vi "comunicación_arduino.vi"() -> ()   [LabVIEW 2026]
uses:
  <vilib>/Instr/_visa.llb/VISA Configure Serial Port (Instr).vi
  <vilib>/Utility/file.llb/Write Delimited Spreadsheet (string).vi
panel:
  out "LED de Histéresis":bool
  in  "Histeresis":dbl
  out "Rango de umbral":bool
  in  "Umbral minimo":dbl
  in  "Umbral maximo":dbl
  in  "Guardar datos":bool
  out "Temperatura minima":dbl
  out "Temperatura maxima":dbl
  out "Waveform Chart":cluster{dbl, dbl, dbl}(graph)
  out "Valor sin filtrar":dbl
  in  "Valor filtrado":bool
  out "Valor filtrado":dbl
  in  "data bits (8)":u16=8 min=5 max=8 step=1
  in  "baud rate (9600)":u32=9600
  out "Dato resivido":string
  in  "Dato a enviar":string
  in  "stop":bool
  in  "Escritura":bool
  in  "Lectura":bool
  in  "VISA resource name":refnum<visa-resource-name>
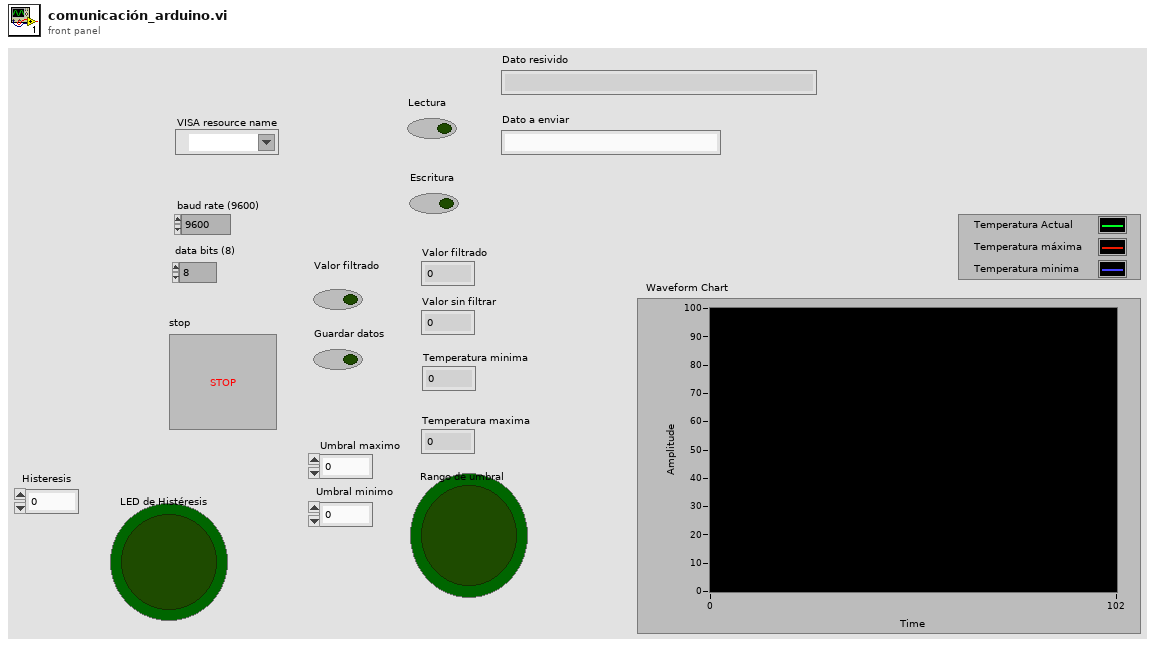
[diagram p1: front panel]
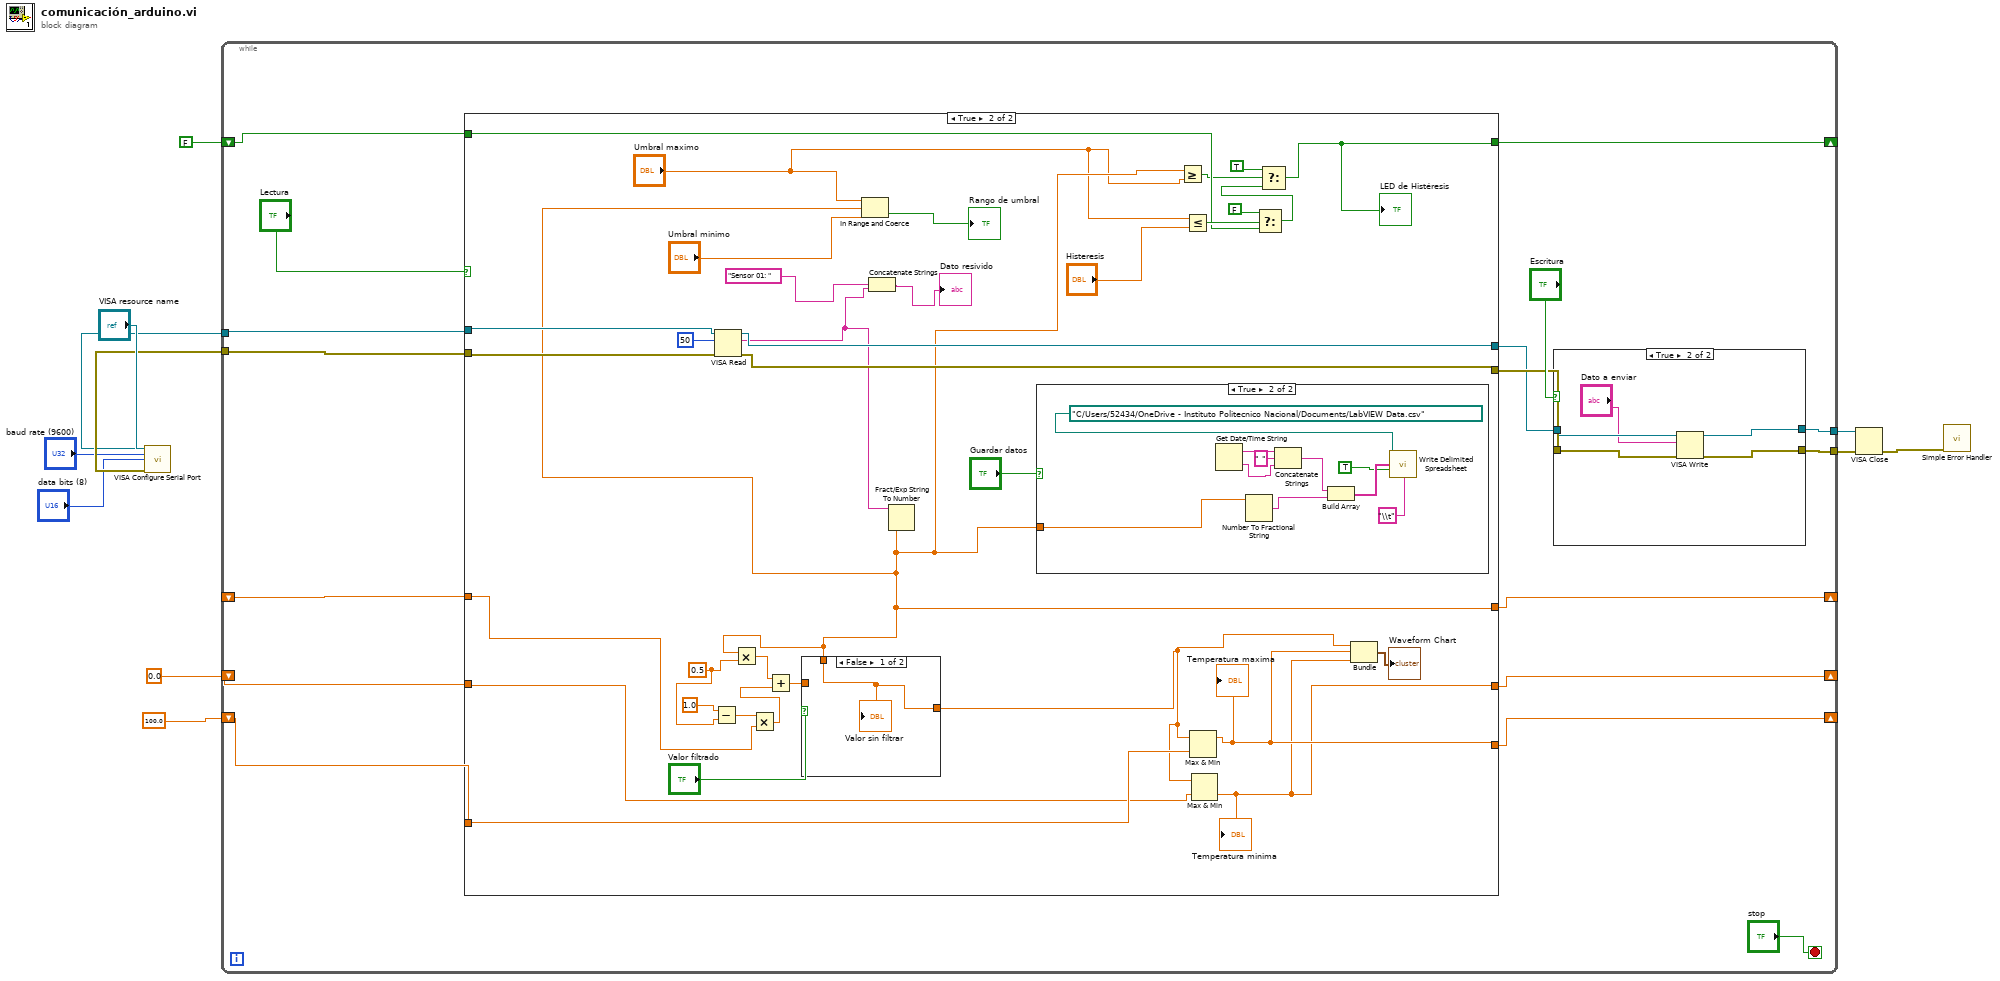
[diagram p0: block diagram]
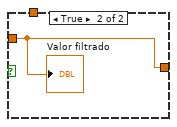
[diagram p5: hidden frame]
diagram:
  n1 = call-poly "VISA Configure Serial Port"("VISA resource name"="VISA resource name", "baud rate (9600)"="baud rate (9600)", "data bits (8)"="data bits (8)") -> ("VISA resource name out"=w9:refnum<visa-resource-name>, "error out"=w10:errorcluster)  [unwired: 11 in]
  n2 = while {
    tunnel: w10 -> [w25]
    tunnel: w9 -> [w22]
    tunnel: [w21] -> w7
    tunnel: [w20] -> w6
    shift-right: [w18] -> _
    shift-left: _ -> [w19]
    shift-right: [w14] -> _
    shift-left: 0.0 -> [w15]
    shift-right: [w16] -> _
    shift-left: 100.0 -> [w17]
    shift-right: [w12] -> _
    shift-left: FALSE -> [w13]
    stop <- "stop" stop-if-true
    n3 = case shown="True" "Lectura" {
      tunnel: w25 -> [w40 w76]
      tunnel: [w40 w75] -> w24
      tunnel: [w41 w74] -> w23
      tunnel: w22 -> [w41 w73]
      tunnel: w19 -> [w39 w67]
      tunnel: [w39 w55] -> w18
      tunnel: w17 -> [w38 w63]
      tunnel: [w38 w61] -> w16
      tunnel: [w37 w60] -> w14
      tunnel: w15 -> [w37 w62]
      tunnel: w13 -> [w36 w50]
      tunnel: [w36 w46] -> w12
      frame False {
      }
      frame True {
        w69 = 0.5 ("y")
        n4 = Subtract(x=1.0, y=w69) -> (x-y=w68:dbl)
        n5 = VISA Read(VISA resource name=w73, byte count=u32 50, error in (no error)=w76) -> (VISA resource name out=w74:refnum<visa-resource-name>, read buffer=w43:string, error out=w75:errorcluster)  [unwired: 1 out]
        n6 = Multiply(x=w68, y=w67) -> (x*y=w66:dbl)
        n7 = Concatenate Strings("Sensor 01: " ("regular expression"), w43) -> (→"Dato resivido":string)
        n8 = Fract/Exp String To Number(string=w43) -> (number=w55:dbl)  [unwired: 3 in, 1 out]
        n9 = Multiply(x=w55, y=w69) -> (x*y=w71:dbl)
        n10 = Add(x=w71, y=w66) -> (x+y=w65:dbl)
        n11 = case shown="False" "Valor filtrado" {
          tunnel: w65 -> [_ w88]
          tunnel: w55 -> [w87 _]
          tunnel: [w87 w88] -> w45
          frame False {
            "Valor sin filtrar" <- w87
          }
          frame True {
            "Valor filtrado" <- w88
          }
        }
        n12 = In Range and Coerce(upper limit="Umbral maximo", x=w55, lower limit="Umbral minimo") -> (In Range?=→"Rango de umbral":bool)  [unwired: 1 out]
        n13 = case shown="True" "Guardar datos" {
          tunnel: w55 -> [_ w83]
          frame False {
          }
          frame True {
            n14 = Get Date/Time String() -> (date string=w86:string, time string=w84:string)  [unwired: 3 in]
            n15 = Number To Fractional String(number=w83) -> (F-format string=w81:string)  [unwired: 3 in]
            n16 = Concatenate Strings(w86, " " ("string"), w84) -> (w82:string)
            n17 = Build Array(w82, w81) -> (w80:string[])
            n18 = call-poly <vilib>:"Write Delimited Spreadsheet.vi"("file path (dialog if empty)"=path "C:/Users/52434/OneDrive - Instituto Politecnico Nacional/Documents/LabVIEW Data.csv", "1D data"=w80, "append to file? (new file:F)"=TRUE, "delimiter (\\t)"="\\t" ("delimiter (\\t)")) -> ()  [unwired: 10 in, 2 out]
          }
        }
        n19 = Greater Or Equal?(x=w55, y="Umbral maximo") -> (x >= y?=w47:bool)
        n20 = Less Or Equal?(x="Umbral maximo", y="Histeresis") -> (x <= y?=w52:bool)
        n21 = Max & Min(x=w45, y=w63) -> (max(x,y)=w61:dbl)  [unwired: 1 out]
        "Temperatura maxima" <- w61
        n22 = Max & Min(x=w45, y=w62) -> (min(x,y)=w60:dbl)  [unwired: 1 out]
        "Temperatura minima" <- w60
        n23 = Select(t=FALSE, s=w52, f=w50) -> (s? t:f=w48:bool)
        n24 = Select(t=TRUE, s=w47, f=w48) -> (s? t:f=w46:bool)
        "LED de Histéresis" <- w46
        n25 = Bundle(w45, w61, w60) -> (→"Waveform Chart":cluster{dbl, dbl, dbl})  [unwired: 1 in]
      }
    }
    n26 = case shown="True" "Escritura" {
      tunnel: w24 -> [w29 w34]
      tunnel: w23 -> [w30 w35]
      tunnel: [w30 w33] -> w21
      tunnel: [w29 w32] -> w20
      frame False {
      }
      frame True {
        n27 = VISA Write(VISA resource name=w35, write buffer="Dato a enviar", error in (no error)=w34) -> (VISA resource name out=w33:refnum<visa-resource-name>, error out=w32:errorcluster)  [unwired: 1 out]
      }
    }
  }
  n28 = VISA Close(VISA resource name=w7, error in (no error)=w6) -> (error out=w8:errorcluster)
  n29 = call <vilib>:"Simple Error Handler.vi"("error in (no error)"=w8) -> ()  [unwired: 4 in, 5 out]
